vi "DE_Update Pareto Indices.vi"(8 "error in (no error)":errorcluster, 11 "State In":T1) -> (0 "error out":errorcluster, 2 "number of feasible":i32, 3 "State Out":T1)   [LabVIEW 2017, in "NI_AAL_GlobalOptimization.lvlib"]
uses:
  <vilib>/gmath/NI_AAL_GlobalOptimization.lvlib
  <vilib>/gmath/GlobalOptimization.llb/DE_State.ctl
  <vilib>/gmath/GlobalOptimization.llb/DE_Population.ctl
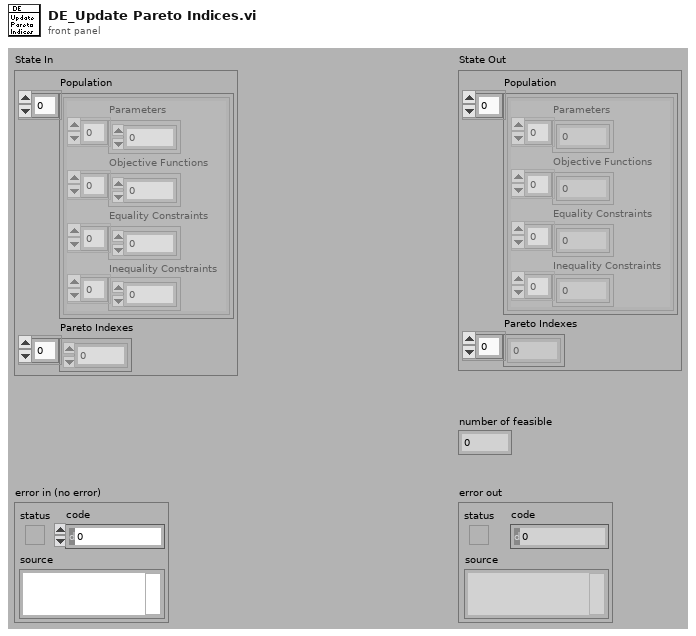
[diagram p1: front panel]
types:
  T1 = typedef "NI_AAL_GlobalOptimization.lvlib/DE_State.ctl" = cluster{"Population":T2[], "Pareto Indexes":i32[]}
  T2 = typedef "NI_AAL_GlobalOptimization.lvlib/DE_Population.ctl" = cluster{"Parameters":dbl[], "Objective Functions":dbl[], "Equality Constraints":dbl[], "Inequality Constraints":dbl[]}
  T3 = typedef "NI_AAL_GlobalOptimization.lvlib/DE_Population Comparison.ctl" = u16
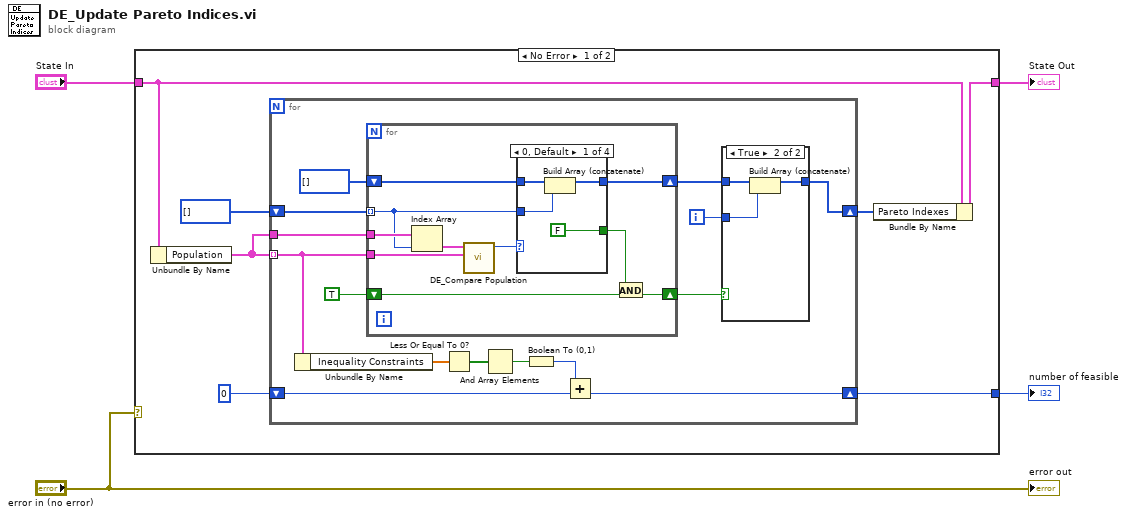
[diagram p0: block diagram]
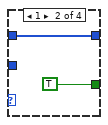
[diagram p3: hidden frame]
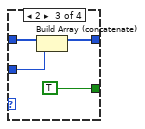
[diagram p4: hidden frame]
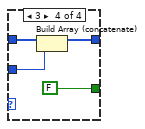
[diagram p5: hidden frame]
diagram:
  n1 = case shown="No Error" "error in (no error)" {
    tunnel: [w11 _] -> w4
    tunnel: "State In" -> [w10 _]
    tunnel: [w9 _] -> w2
    frame No Error {
      n2 = Unbundle By Name(w10) -> ("Population"=w8:T2[])
      n3 = for {
        tunnel: w8 -> [w12] mode=indexing
        tunnel: w8 -> [w26]
        shift-right: [w20] -> w6
        shift-left: i32[] [] ("pareto indices") -> [w25]
        shift-right: [w13] -> w9
        shift-left: 0 -> [w14]
        i -> [w21]
        n4 = Unbundle By Name(w12) -> ("Inequality Constraints"=w18:dbl[])
        n5 = for {
          tunnel: w26 -> [w39]
          tunnel: w25 -> [w38] mode=indexing
          shift-right: [w36] -> w23
          shift-left: i32[] [] -> [w37]
          shift-right: [w34] -> w22
          shift-left: TRUE -> [w33]
          tunnel: w12 -> [w31]
          n6 = Index Array(array=w39, index=w38) -> (element=w32:T2)
          n7 = call <vilib>:"DE_Compare Population.vi"("Population B"=w31, "Population A"=w32) -> ("population comparison"=w40:T3)  [unwired: 8 in, 1 out]
          n8 = case shown="0, Default" w40 {
            tunnel: w38 -> [w43 _ w48 w52]
            tunnel: w37 -> [w44 w45 w49 w53]
            tunnel: [w42 w45 w47 w51] -> w36
            tunnel: [FALSE TRUE TRUE FALSE] -> w35
            frame 0, Default {
              n9 = Build Array (concatenate)(w44, w43) -> (w42:i32[])
            }
            frame 1 {
            }
            frame 2 {
              n10 = Build Array (concatenate)(w49, w48) -> (w47:i32[])
            }
            frame 3 {
              n11 = Build Array (concatenate)(w53, w52) -> (w51:i32[])
            }
          }
          n12 = And(x=w35, y=w33) -> (x .and. y?=w34:bool)
        }
        n13 = Less Or Equal To 0?(x=w18) -> (x <= 0?=w17:bool[])
        n14 = And Array Elements(Boolean array=w17) -> (logical AND=w16:bool)
        n15 = Boolean To (0,1)(Boolean=w16) -> (0, 1=w15:i16)
        n16 = Add(x=w15, y=w14) -> (x+y=w13:i32)
        n17 = case shown="True" w22 {
          tunnel: w23 -> [w27 w30]
          tunnel: w21 -> [_ w29]
          tunnel: [w27 w28] -> w20
          frame False {
          }
          frame True {
            n18 = Build Array (concatenate)(w30, w29) -> (w28:i32[])
          }
        }
      }
      n19 = Bundle By Name(cluster=w10, "Pareto Indexes"=w6) -> (w11:T1)
    }
    frame Error {
    }
  }
  "State Out" <- w4
  "number of feasible" <- w2
  "error out" <- "error in (no error)"
